vi "LKIF2_StartMeasure.vi"(8 "error in (no error)":errorcluster) -> (0 "error out":errorcluster)   [LabVIEW 2013, in "Keyence LK-G5000.lvlib"]
uses:
  <instrlib>/Keyence LK-G5000/Keyence LK-G5000.lvlib
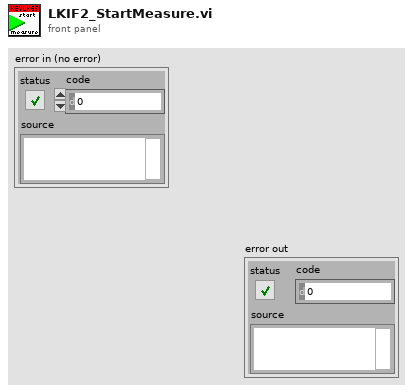
[diagram p1: front panel]
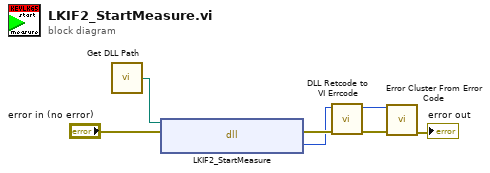
[diagram p0: block diagram]
diagram:
  n1 = call <instrlib>:"Get DLL Path.vi"() -> ("DLL Path"=w7:path)  [unwired: 1 in]
  n2 = dll-call lib="C:/Program Files (x86)/National Instruments/LabVIEW 2013/instr.lib/Keyence LK-G5000/LKIF2.dll" fn="LKIF2_StartMeasure"(path in=w7, error in="error in (no error)") -> (error out=w5:errorcluster, "RC"=w4:i32)  [unwired: 1 in, 1 out]
  n3 = call <instrlib>:"DLL Retcode to VI Errcode.vi"("error in (no error)"=w5, "DLL Retcode"=w4) -> ("error out"=w3:errorcluster, "VI Errcode"=w6:i32)  [unwired: 8 in]
  n4 = call <vilib>:"Error Cluster From Error Code.vi"("error in (no error)"=w3, "error code (0)"=w6) -> ("error out"=→"error out":errorcluster)  [unwired: 7 in]
